vi "Run.vi"(8 "error in (no error)":errorcluster, 9 "Time Ratio used":dbl, 10 "Maze (0: Empty, -1: Enemy. >0: Teammate":i32[][](array[numeric]), 11 "Line Dancer in":refnum<class "Fractal.lvclass">) -> (0 "error out":errorcluster, 1 "Direction":T1, 2 "Action":T2, 3 "Line Dancer out":refnum<class "Fractal.lvclass">, 4 "Replicated":refnum<class "Square.lvclass">)   [LabVIEW 2015, in "Fractal.lvclass"]
uses:
  Fractal.lvclass
  Type Defs/Action Enum.ctl
  Type Defs/Direction Enum.ctl
  Square/Square.lvclass
  Fractal.lvclass/Fractal.ctl
  Line Dancer Type.ctl
  SubVIs/Read-Only Globals.vi
  Type Defs/SB Type Defs.lvlib
  Common/Common.lvlib
panel:
  # "NOTICE - YOU MUST NOT REMOVE THIS NOTICE. PER THE FOLLOWING LICENSE, YOU MAY REPRODUCE THIS SOFTWARE PROVIDED YOU FOLLOW THE TERMS\nOF THE LICENSE.\n\n---BEGIN BSD LICENSE (http://opensource.org/licenses/BSD-2-Clause)---\nCopyright (c) 2015, Endigit, Inc. <robert@endigit.com>\nAll rights reserved.\n\nRedistribution and use in source and binary forms, with or without modification, are permitted provided that the following conditions are met:\n\n1. Redistributions of source code must retain the above copyright notice, this list of conditions and the following disclaimer.\n\n2. Redistributions in binary form must reproduce the above copyright notice, this list of conditions and the following disclaimer in the documentation and/or other \nmaterials provided with the distribution.\n\nTHIS SOFTWARE IS PROVIDED BY THE COPYRIGHT HOLDERS AND CONTRIBUTORS \"AS IS\" AND ANY EXPRESS OR IMPLIED WARRANTIES, INCLUDING, BUT NOT \nLIMITED TO, THE IMPLIED WARRANTIES OF MERCHANTABILITY AND FITNESS FOR A PARTICULAR PURPOSE ARE DISCLAIMED. IN NO EVENT SHALL THE COPYRIGHT \nHOLDER OR CONTRIBUTORS BE LIABLE FOR ANY DIRECT, INDIRECT, INCIDENTAL, SPECIAL, EXEMPLARY, OR CONSEQUENTIAL DAMAGES (INCLUDING, BUT NOT \nLIMITED TO, PROCUREMENT OF SUBSTITUTE GOODS OR SERVICES; LOSS OF USE, DATA, OR PROFITS; OR BUSINESS INTERRUPTION) HOWEVER CAUSED AND ON \nANY THEORY OF LIABILITY, WHETHER IN CONTRACT, STRICT LIABILITY, OR TORT (INCLUDING NEGLIGENCE OR OTHERWISE) ARISING IN ANY WAY OUT OF THE USE \nOF THIS SOFTWARE, EVEN IF ADVISED OF THE POSSIBILITY OF SUCH DAMAGE.\n---END BSD LICENSE---"
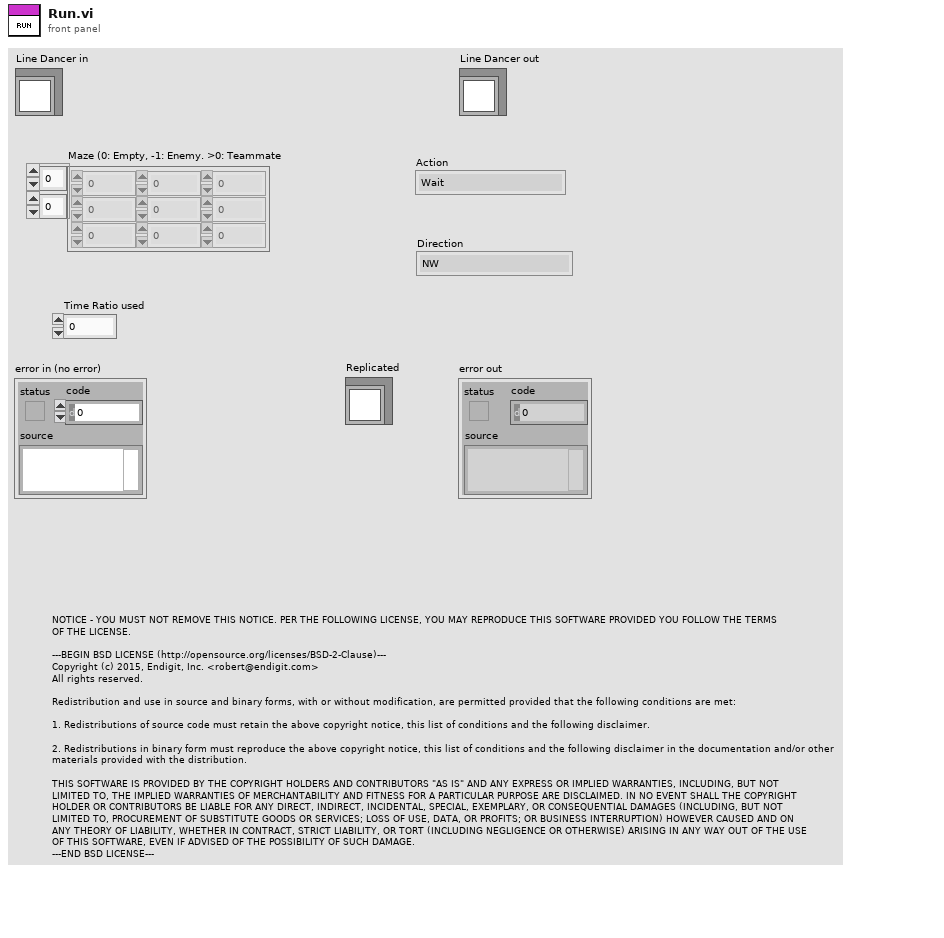
[diagram p1: front panel]
types:
  T1 = typedef "SB Type Defs.lvlib/Direction Enum.ctl" = enum16{"NW", "N", "NE", "E", "SE", "S", "SW", "W"}
  T2 = typedef "SB Type Defs.lvlib/Action Enum.ctl" = enum16{"Wait", "Move", "Attack", "Replicate"}
  T3 = typedef "Fractal.lvclass/Line Dancer Type.ctl" = enum16{"Top", "Bottom", "Start"}
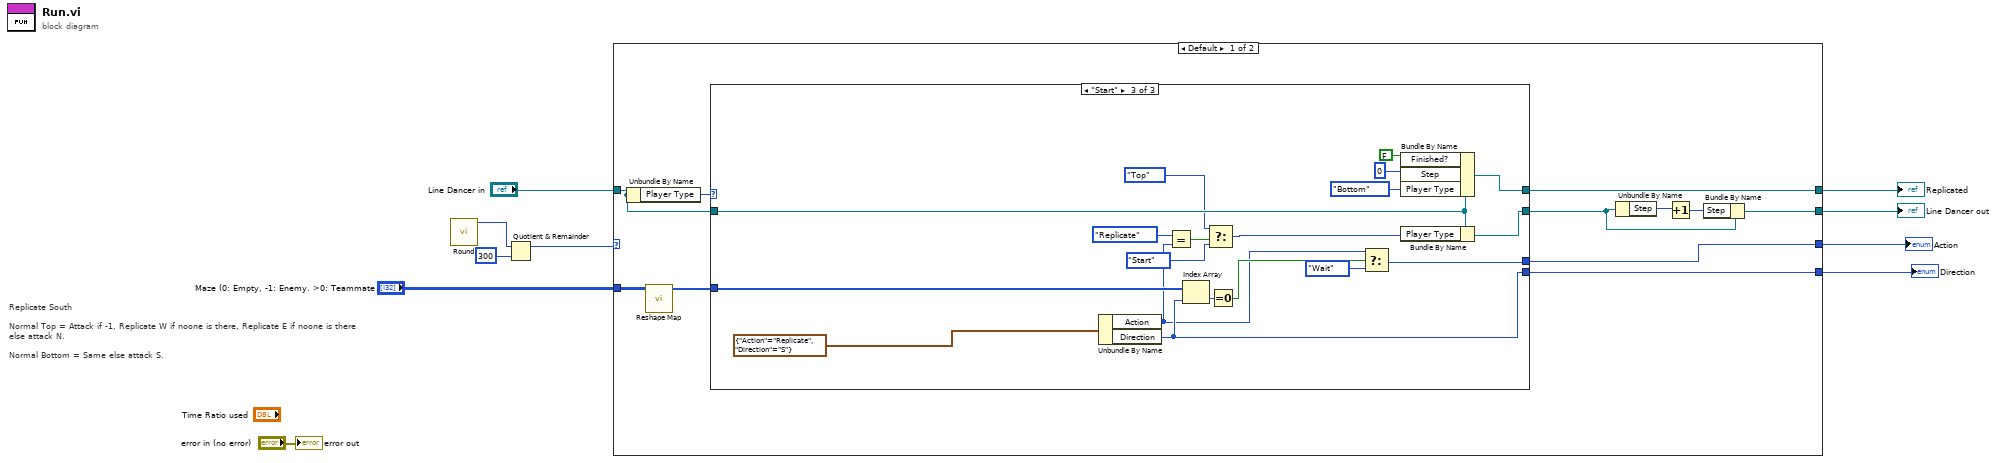
[diagram p0: block diagram]
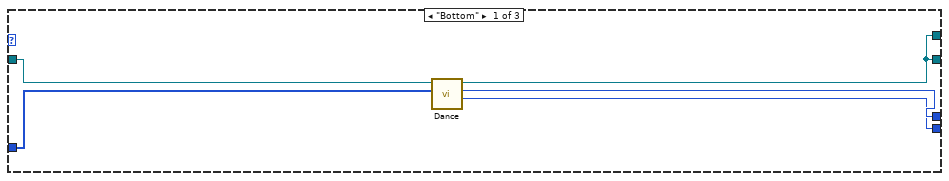
[diagram p2: hidden frame]
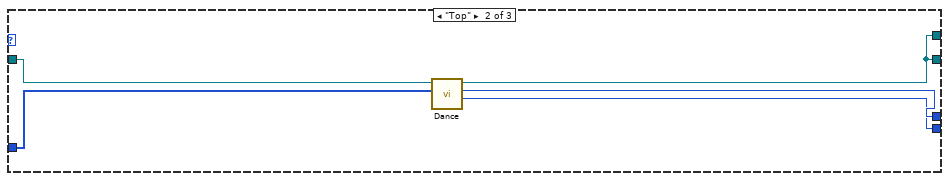
[diagram p3: hidden frame]
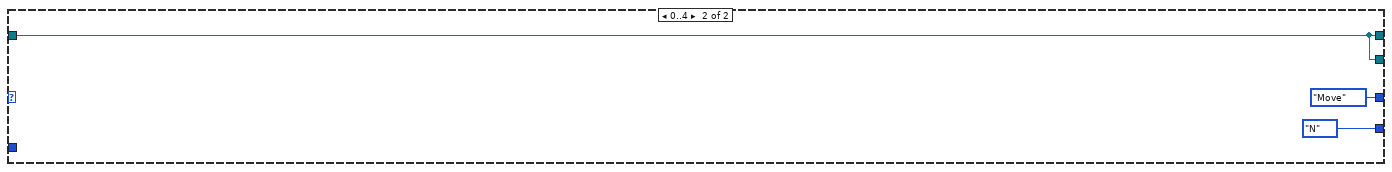
[diagram p4: hidden frame]
diagram:
  # "Replicate South\n\nNormal Top = Attack if -1, Replicate W if noone is there, Replicate E if noone is there\nelse attack N.\n\nNormal Bottom = Same else attack S."
  n1 = call "Round.vi"() -> ("Round"=w3:i32)  [unwired: 11 in]
  n2 = Quotient & Remainder(x=w3, y=300) -> (x-y*floor(x/y)=w1:i32)  [unwired: 1 out]
  n3 = case shown="Default" w1 {
    tunnel: [w21 Action_Enum."Move" ("f")] -> w9
    tunnel: [w20 Direction_Enum."N" ("Direction")] -> w8
    tunnel: "Maze (0: Empty, -1: Enemy. >0: Teammate" -> [w19 _]
    tunnel: "Line Dancer in" -> [w16 w53]
    tunnel: [w12 w53] -> w5
    tunnel: [w11 w53] -> w4
    frame Default {
      n4 = Unbundle By Name(w16) -> ("Player Type"=w17:T3)
      n5 = call "Reshape Map.vi"("Maze (0: Empty, -1: Enemy. >0: Teammate"=w19) -> ("Map"=w18:i32[])  [unwired: 9 in, 1 out]
      n6 = case shown="\"Start\"" w17 {
        tunnel: [w26 w31 w42] -> w21
        tunnel: [w25 w30 w45] -> w20
        tunnel: w18 -> [w24 w29 w46]
        tunnel: [w22 w27 w49] -> w11
        tunnel: [w22 w27 w48] -> w13
        tunnel: w16 -> [w23 w28 w44]
        frame "Bottom" {
          n7 = call "Dance.vi"("Map"=w24, "Line Dancer in"=w23) -> ("index of element"=w25:i32, "Action"=w26:T2, "Line Dancer out"=w22:refnum<class "Fractal.lvclass">)  [unwired: 7 in]
        }
        frame "Top" {
          n8 = call "Dance.vi"("Map"=w29, "Line Dancer in"=w28) -> ("index of element"=w30:i32, "Action"=w31:T2, "Line Dancer out"=w27:refnum<class "Fractal.lvclass">)  [unwired: 7 in]
        }
        frame "Start" {
          n9 = Unbundle By Name(cluster{"Action":T2, "Direction":T1} {"Action"=enum."Replicate", "Direction"=enum."S"}) -> ("Action"=w38:T2, "Direction"=w45:T1)
          n10 = Equal?(x=Action_Enum."Replicate", y=w38) -> (x = y?=w39:bool)
          n11 = Index Array(array=w46, index=w45) -> (element=w43:i32)
          n12 = Select(t=Line_Dancer_Type."Top" ("Player Type"), s=w39, f=Line_Dancer_Type."Start" ("Player Type")) -> (s? t:f=w34:T3)
          n13 = Equal To 0?(x=w43) -> (x = 0?=w41:bool)
          n14 = Select(t=w38, s=w41, f=Action_Enum."Wait") -> (s? t:f=w42:T2)
          n15 = Bundle By Name(cluster=w44, "Finished?"=FALSE, "Step"=0, "Player Type"=Line_Dancer_Type."Bottom") -> (w49:refnum<class "Fractal.lvclass">)
          n16 = Bundle By Name(cluster=w44, "Player Type"=w34) -> (w48:refnum<class "Fractal.lvclass">)
        }
      }
      n17 = Unbundle By Name(w13) -> ("Step"=w15:i32)
      n18 = Increment(x=w15) -> (x+1=w14:i32)
      n19 = Bundle By Name(cluster=w13, "Step"=w14) -> (w12:refnum<class "Fractal.lvclass">)
    }
    frame 0..4 {
    }
  }
  "Line Dancer out" <- w5
  "Action" <- w9
  "Direction" <- w8
  "Replicated" <- w4
  "error out" <- "error in (no error)"
